vi "list available classifications.vi"() -> (3 "supported types":T1[](array[typedef]))   [LabVIEW 2013, in "TBM channel.lvclass"]
uses:
  TBM channel.lvclass
  channel classification.ctl
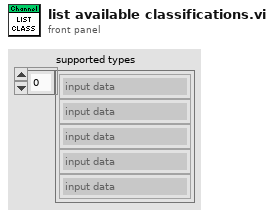
[diagram p1: front panel]
types:
  T1 = typedef "TBM channel.lvclass/channel classification.ctl" = enum16{"input data", "output data", "processing parameter", "processing result"}
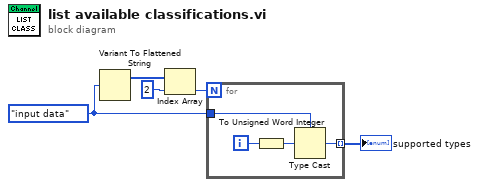
[diagram p0: block diagram]
diagram:
  w3 = channel_classification."input data" ("channel classification")
  n1 = Variant To Flattened String(Variant=w3) -> (1:w5:i16[])  [unwired: 1 out]
  n2 = Index Array(array=w5, index=2) -> (element=w1:i16)
  n3 = for {
    N: w1 -> [_]
    tunnel: w3 -> [w8]
    tunnel: [w7] -> w2 mode=indexing
    i -> [w6]
    n4 = To Unsigned Word Integer(number=w6) -> (unsigned 16bit integer=w9:u16)
    n5 = Type Cast(type=w8, x=w9) -> (*(type *) &x=w7:T1)
  }
  "supported types" <- w2
